vi "Fdx Stop (Tx).vi"(8 "error in":errorcluster, 10 "Force Stop?":bool, 11 "InstrumentHandle_port in":u32) -> (0 "error out":errorcluster, 3 "InstrumentHandle_port out":u32)   [LabVIEW 2020, in "AIM664LV.lvlib"]
uses:
  AIM664LV.lvlib
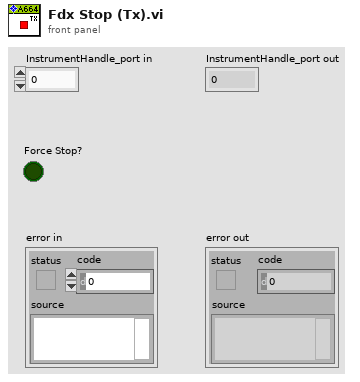
[diagram p1: front panel]
types:
  T1 = cluster{"StartMode":i32, "Count":u32, "Sign":i32, "Day":u32, "Hour":u32, "Min":u32, "Second":u32, "MilliSec":u32, "MicroSec":u32, "ExtendedStopMode":i32, "TransmitTime":u32}
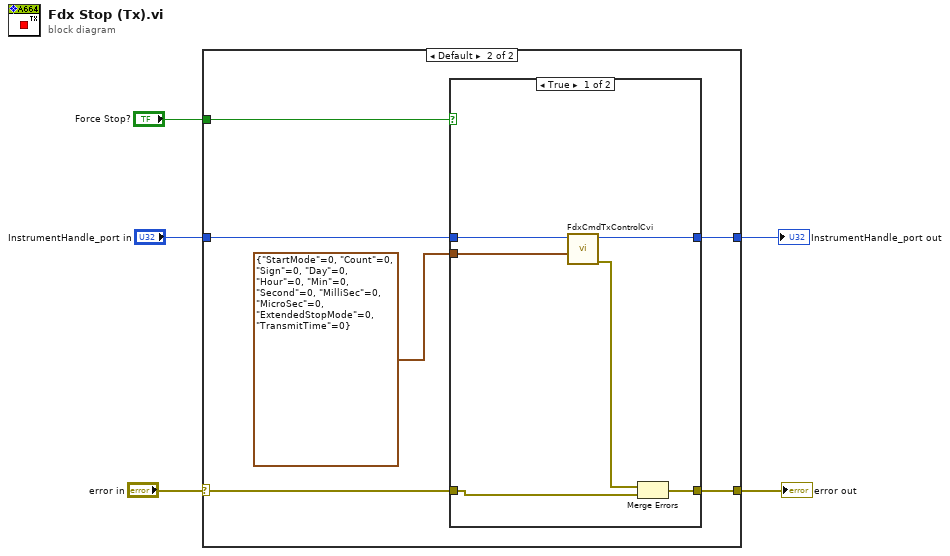
[diagram p0: block diagram]
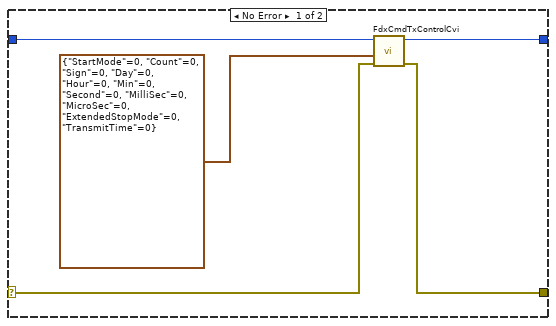
[diagram p2: hidden frame]
diagram:
  n1 = case shown="Default" "error in" {
    selector: "error in" -> [w8 w14]
    tunnel: [w10 w16] -> w5
    tunnel: "Force Stop?" -> [_ w13]
    tunnel: [w7 w12] -> w2
    tunnel: "InstrumentHandle_port in" -> [w6 w11]
    frame No Error {
      n2 = call "FdxCmdTxControlCvi.vi"("error in"=w8, "TxControl"=T1 {"StartMode"=0, "Count"=0, "Sign"=0, "Day"=0, "Hour"=0, "Min"=0, "Second"=0, "MilliSec"=0, "MicroSec"=0, "ExtendedStopMode"=0, "TransmitTime"=0} ("TxControl 2"), "InstrumentHandle_port"=w6) -> ("error out"=w10:errorcluster, "InstrumentHandle_port"=w7:u32)  [unwired: 7 in]
    }
    frame Default {
      n3 = case shown="True" w13 {
        tunnel: [w22 w23] -> w12
        tunnel: [w18 w24] -> w16
        tunnel: T1 {"StartMode"=0, "Count"=0, "Sign"=0, "Day"=0, "Hour"=0, "Min"=0, "Second"=0, "MilliSec"=0, "MicroSec"=0, "ExtendedStopMode"=0, "TransmitTime"=0} ("TxControl 2") -> [w20 _]
        tunnel: w14 -> [w17 w24]
        tunnel: w11 -> [w19 w23]
        frame True {
          n4 = call "FdxCmdTxControlCvi.vi"("TxControl"=w20, "InstrumentHandle_port"=w19) -> ("error out"=w21:errorcluster, "InstrumentHandle_port"=w22:u32)  [unwired: 8 in]
          n5 = Merge Errors(w21, w17) -> (w18:errorcluster)
        }
        frame False {
        }
      }
    }
  }
  "error out" <- w5
  "InstrumentHandle_port out" <- w2
